vi "Main Page.vi"(8 "error in (no error)":errorcluster, 11 "Node Ptr":T1 format="%.0x") -> (0 "error out":errorcluster)   [LabVIEW 2021, in "Large Number Operation System Explorer.lvlib"]
uses:
  Large Number Operation System Explorer.lvlib
  <vilib>/NI VeriStand/Custom Device API/Custom Device Item Ref.ctl
  <vilib>/NI VeriStand/Custom Device API/Get Item Property (U16).vi
  <vilib>/NI VeriStand/Custom Device API/Set Item Property (U16).vi
  <vilib>/NI VeriStand/Custom Device API/Custom Device API.lvlib
  <vilib>/NI VeriStand/Custom Device API/Set Item Property (String).vi
  <vilib>/NI VeriStand/Custom Device API/Get Item Property (String).vi
panel:
  in  "Address":string
  in  "Async Timeout (ms)":u16
  out "Version":string
  in  "SHDocVw.IWebBrowser":refnum<k7>(container)
  in  "Specific Header":cluster{"Section Name":string}={"Section Name"="gRPC Client Settings"}
  in  "General Header":cluster{"Section Name":string}={"Section Name"="General Custom Device Settings"}
  in  "Description":string
  in  "Name":string
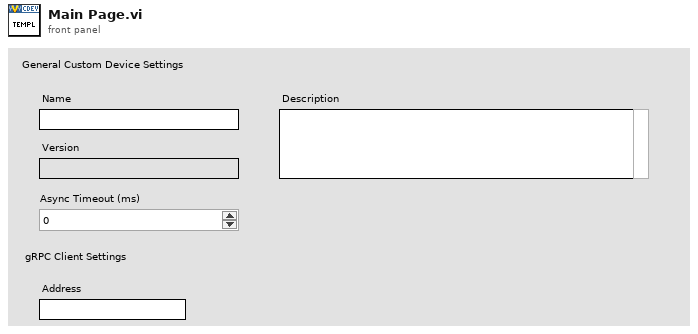
[diagram p1: front panel]
types:
  T1 = typedef "Custom Device API.lvlib/Custom Device Item Ref.ctl" = u64
  T2 = typedef "Custom Device API.lvlib/Custom Device Item Info.ctl" = cluster{"Name":string, "Is Channel":bool, "GUID":string, "Is Waveform":bool}
  T3 = typedef "Custom Device API.lvlib/Custom Device Commands.ctl" = enum16{"Default", "Item renamed", "Shutdown", "Dynamic button pressed"}
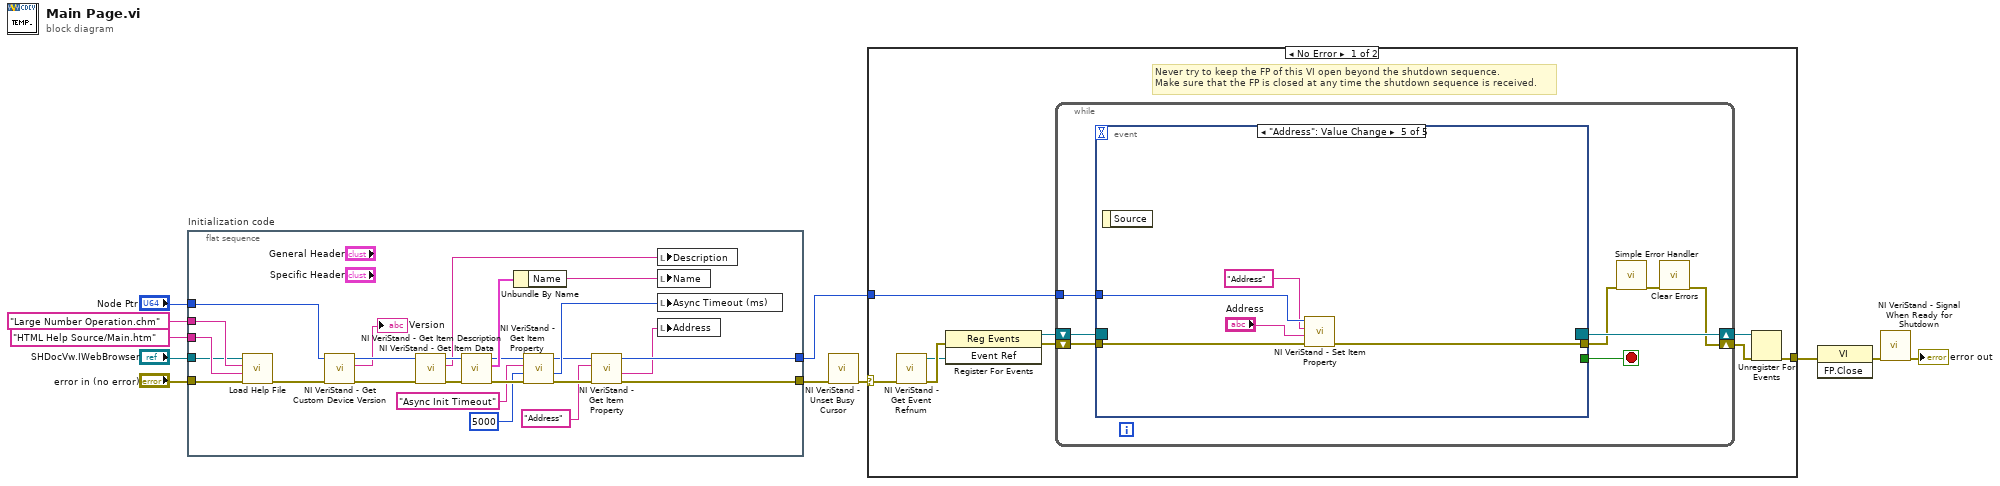
[diagram p0: block diagram]
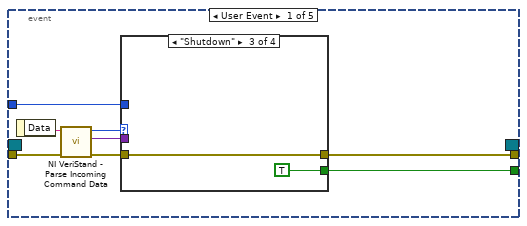
[diagram p2: hidden frame]
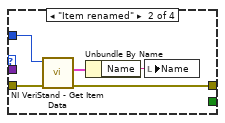
[diagram p4: hidden frame]
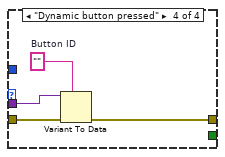
[diagram p5: hidden frame]
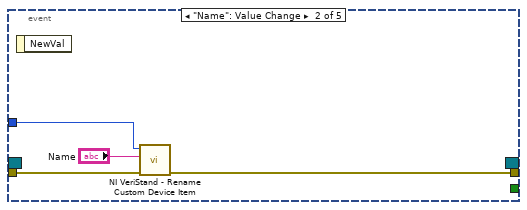
[diagram p6: hidden frame]
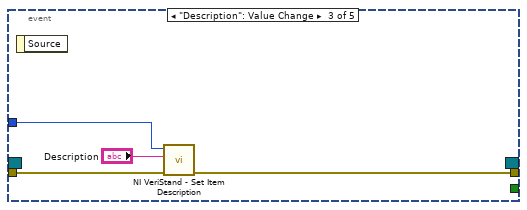
[diagram p7: hidden frame]
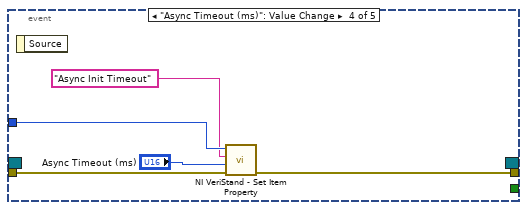
[diagram p8: hidden frame]
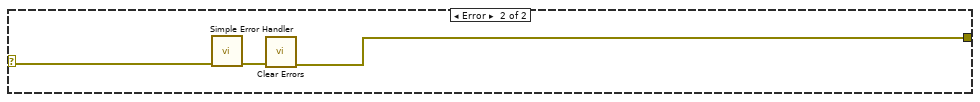
[diagram p9: hidden frame]
diagram:
  n1 = flat-sequence "Initialization code" {
    tunnel: "error in (no error)" -> [w27]
    tunnel: "Node Ptr" -> [w33]
    tunnel: [w15] -> w7
    tunnel: [w16] -> w4
    tunnel: "SHDocVw.IWebBrowser" -> [w23]
    tunnel: "HTML Help Source/Main.htm" ("HTML File") -> [w24]
    tunnel: "Large Number Operation.chm" ("CD_CHM_FileName") -> [w25]
    frame #0 {
      n2 = call "Load Help File.vi"("error in (no error)"=w27, "HTML File to Load"=w24, "Main CHM File"=w25, "Browser"=w23) -> ("error out"=w26:errorcluster)  [unwired: 7 in]
      n3 = call <vilib>:"NI VeriStand - Get Custom Device Version.vi"("error in (no error)"=w26, "Device Ref in"=w33) -> ("error out"=w32:errorcluster, "Value"=→"Version":string, "Device Ref out"=w31:T1)  [unwired: 7 in]
      n4 = call <vilib>:"NI VeriStand - Get Item Description.vi"("error in (no error)"=w32, "Item Ref in"=w31) -> ("error out"=w35:errorcluster, "Description"=w28:string, "Item Ref out"=w36:T1)  [unwired: 7 out]
      n5 = call <vilib>:"NI VeriStand - Get Item Data.vi"("error in (no error)"=w35, "Item Ref in"=w36) -> ("error out"=w22:errorcluster, "Item Info"=w34:T2, "Item Ref out"=w21:T1)  [unwired: 7 out]
      n6 = Unbundle By Name(w34) -> ("Name"=w29:string)
      n7 = call-poly <vilib>:"NI VeriStand - Get Item Property.vi"("error in (no error)"=w22, "Default Value"=u16 5000, "Property Name"="Async Init Timeout", "Item Ref in"=w21) -> ("error out"=w14:errorcluster, "Value"=w20:u16, "Item Ref out"=w17:T1)  [unwired: 4 in, 1 out]
      n8 = call-poly <vilib>:"NI VeriStand - Get Item Property.vi"("error in (no error)"=w14, "Property Name"="Address", "Item Ref in"=w17) -> ("error out"=w15:errorcluster, "Value"=w13:string, "Item Ref out"=w16:T1)  [unwired: 5 in, 1 out]
      n9 = local write "Description"(w28) -> ()
      n10 = local write "Name"(w29) -> ()
      n11 = local write "Async Timeout (ms)"(w20) -> ()
      n12 = local write "Address"(w13) -> ()
    }
  }
  n13 = call <vilib>:"NI VeriStand - Unset Busy Cursor.vi"("error in (no error)"=w7) -> ("error out"=w6:errorcluster)  [unwired: 10 out]
  n14 = case shown="No Error" w6 {
    selector: w6 -> [w37 w94]
    tunnel: [w42 w92] -> w11
    tunnel: w4 -> [w38 _]
    frame No Error {
      # "Never try to keep the FP of this VI open beyond the shutdown sequence.\nMake sure that the FP is closed at any time the shutdown sequence is received."
      n15 = call <vilib>:"NI VeriStand - Get Event Refnum.vi"("error in (no error)"=w37) -> ("error out"=w45:errorcluster, "Event Ref"=w41:refnum<user-event>)  [unwired: 9 out]
      n16 = register-events(error in=w45, w41) -> (reference out=w39:refnum<event-registration>, error out=w40:errorcluster)  [unwired: 1 in]
      n17 = while {
        tunnel: w38 -> [w49]
        shift-right: [w46] -> w43
        shift-left: w40 -> [w52]
        shift-right: [w53] -> w44
        shift-left: w39 -> [w51]
        stop <- w50 stop-if-true
        n18 = event shown="[4] \"Address\": Value Change" {
          selector: w51 -> [_ _ _ _ _]
          dyn-events: [_ _ _ _ _] -> w53
          timeout: _ -> [_ _ _ _ _]
          tunnel: w52 -> [w61 w77 w80 w86 w91]
          tunnel: [w57 _ _ _ _] -> w50
          tunnel: [w56 w76 w79 w83 w89] -> w48
          tunnel: w49 -> [w55 w75 w81 w85 w90]
          event User Event {
            n19 = event-data() -> ("Data"=w60:string)  [unwired: 1 out]
            n20 = call <vilib>:"NI VeriStand - Parse Incoming Command Data.vi"("error in (no error)"=w61, "Incoming data"=w60) -> ("error out"=w59:errorcluster, "Outgoing data"=w54:variant, "Action"=w58:T3)  [unwired: 7 out]
            n21 = case shown="\"Shutdown\"" w58 {
              tunnel: w59 -> [w62 w67 w68 w73]
              tunnel: [_ _ TRUE _] -> w57
              tunnel: [w62 w64 w68 w70] -> w56
              tunnel: w55 -> [_ w66 _ _]
              tunnel: w54 -> [_ _ _ w72]
              frame "Default", Default {
              }
              frame "Item renamed" {
                n22 = call <vilib>:"NI VeriStand - Get Item Data.vi"("error in (no error)"=w67, "Item Ref in"=w66) -> ("error out"=w64:errorcluster, "Item Info"=w65:T2)  [unwired: 8 out]
                n23 = Unbundle By Name(w65) -> ("Name"=w63:string)
                n24 = local write "Name"(w63) -> ()
              }
              frame "Shutdown" {
              }
              frame "Dynamic button pressed" {
                w71 = ""  # Button ID
                n25 = Variant To Data(error in=w73, type=w71, Variant=w72) -> (error out=w70:errorcluster)  [unwired: 1 out]
              }
            }
          }
          event "Name": Value Change {
            n26 = event-data() -> ()  [unwired: 2 out]
            n27 = call <vilib>:"NI VeriStand - Rename Custom Device Item.vi"("error in (no error)"=w77, "New Name"="Name", "Item Ref in"=w75) -> ("error out"=w76:errorcluster)  [unwired: 1 in, 7 out]
          }
          event "Description": Value Change {
            n28 = event-data() -> ()  [unwired: 2 out]
            n29 = call <vilib>:"NI VeriStand - Set Item Description.vi"("error in (no error)"=w80, "Description"="Description", "Item Ref in"=w81) -> ("error out"=w79:errorcluster)  [unwired: 8 out]
          }
          event "Async Timeout (ms)": Value Change {
            n30 = event-data() -> ()  [unwired: 2 out]
            n31 = call-poly <vilib>:"NI VeriStand - Set Item Property.vi"("error in (no error)"=w86, "Value"="Async Timeout (ms)", "Property Name"="Async Init Timeout", "Item Ref in"=w85) -> ("error out"=w83:errorcluster)  [unwired: 5 in, 2 out]
          }
          event "Address": Value Change {
            n32 = event-data() -> ()  [unwired: 2 out]
            n33 = call-poly <vilib>:"NI VeriStand - Set Item Property.vi"("error in (no error)"=w91, "Value"="Address", "Property Name"="Address", "Item Ref in"=w90) -> ("error out"=w89:errorcluster)  [unwired: 5 in, 2 out]
          }
        }
        n34 = call <vilib>:"Simple Error Handler.vi"("error in (no error)"=w48) -> ("error out"=w47:errorcluster)  [unwired: 1 in, 7 out]
        n35 = call <vilib>:"Clear Errors.vi"("error in (no error)"=w47) -> ("error out"=w46:errorcluster)  [unwired: 1 in, 5 out]
      }
      n36 = Unregister For Events(event registration refnum=w44, error in=w43) -> (error out=w42:errorcluster)
    }
    frame Error {
      n37 = call <vilib>:"Simple Error Handler.vi"("error in (no error)"=w94) -> ("error out"=w93:errorcluster)  [unwired: 1 in, 7 out]
      n38 = call <vilib>:"Clear Errors.vi"("error in (no error)"=w93) -> ("error out"=w92:errorcluster)  [unwired: 1 in, 5 out]
    }
  }
  n39 = invoke class="VI" method="FP.Close"(error in=w11) -> (error out=w10:errorcluster)  [unwired: 2 in, 2 out]
  n40 = call <vilib>:"NI VeriStand - Signal When Ready for Shutdown.vi"("error in (no error)"=w10) -> ("error out"=→"error out":errorcluster)  [unwired: 10 out]
